vi "Read Property.vi"(8 "error in (no error)":errorcluster, 11 "2D Plot.lvclass in":refnum<class "2D Plot.lvclass">) -> (0 "error out":errorcluster, 2 "XY Graph Property Cluster":T1, 3 "2D Plot.lvclass out":refnum<class "2D Plot.lvclass">)   [LabVIEW 2020, in "2D Plot.lvclass"]
uses:
  <vilib>/Math Plots/2D Math Plots/2D Plot/2D Plot/2D Plot.lvclass
  <vilib>/Math Plots/2D Math Plots/2D Plot/2D Plot/Typedef/Property Cluster.ctl
  <vilib>/Math Plots/2D Math Plots/2D Plot/2D Plot/Typedef/Graph General Property.ctl
  <vilib>/Math Plots/2D Math Plots/2D Plot/2D Plot/Typedef/Scale Array.ctl
  <vilib>/Math Plots/2D Math Plots/2D Plot/2D Plot/Typedef/Scale Cluster.ctl
  <vilib>/Utility/miscctls.llb/LVOffsetAndMultiplierTypeDef.ctl
  <vilib>/Math Plots/2D Math Plots/2D Plot/2D Plot/Typedef/Cursor Property.ctl
  <vilib>/Utility/miscctls.llb/LVCursorListTypeDef.ctl
  <vilib>/Utility/miscctls.llb/LVAnnotationListTypeDef.ctl
  <vilib>/Math Plots/2D Math Plots/2D Plot/2D Plot/2D Plot.lvclass/2D Plot.ctl
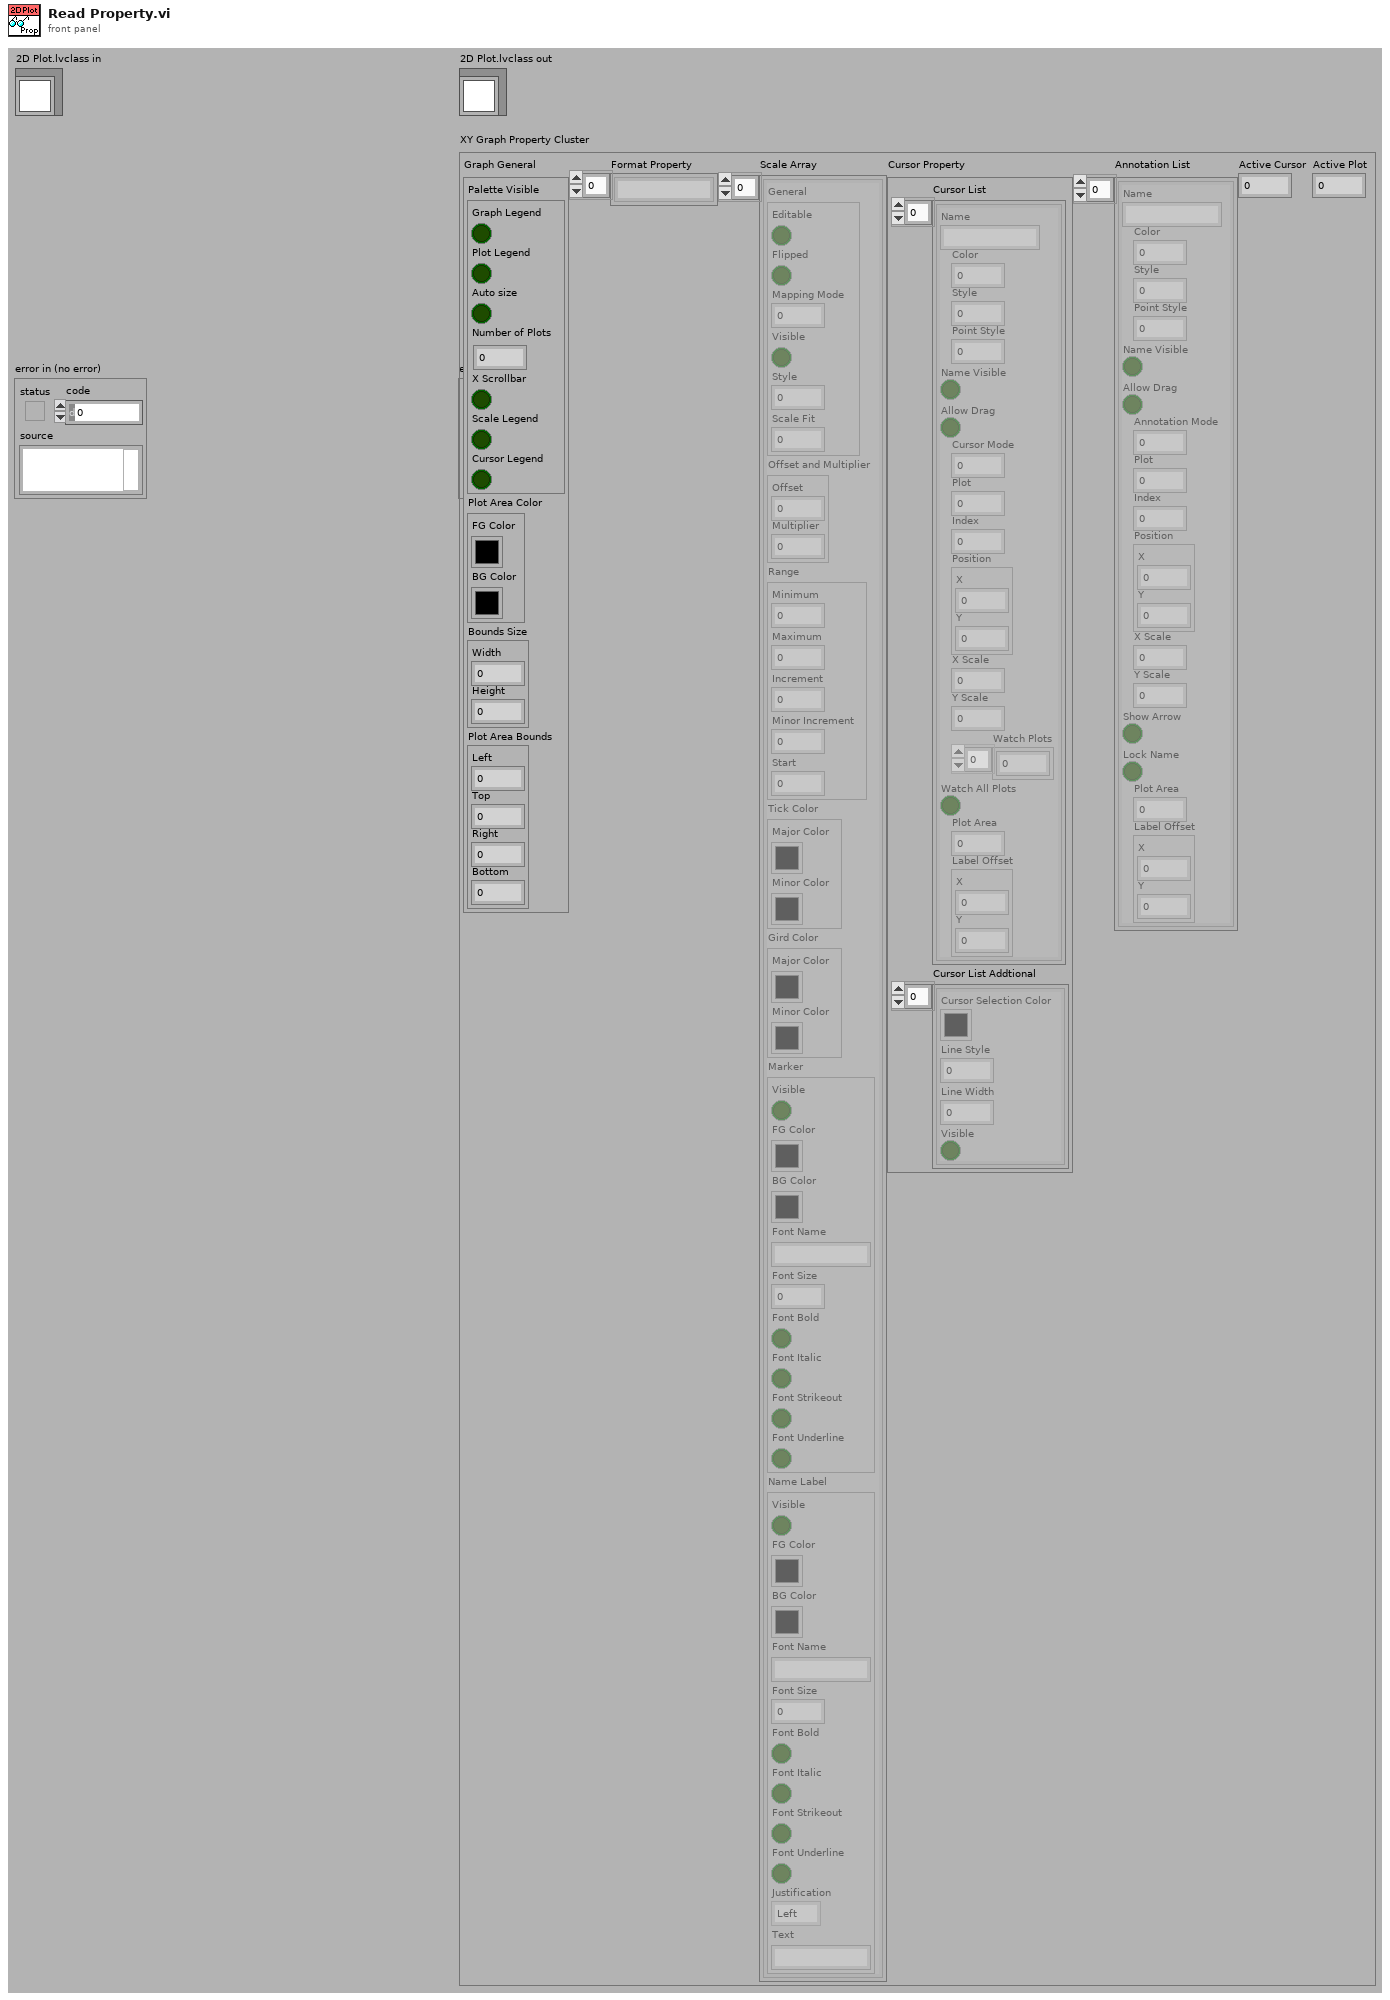
[diagram p1: front panel]
types:
  T1 = typedef "2D Plot.lvclass/Property Cluster.ctl" = cluster{"Graph General":T2, "Format Property":string[], "Scale Array":T3, "Cursor Property":T6, "Annotation List":T8, "Active Cursor":i32, "Active Plot":i32}
  T2 = typedef "2D Plot.lvclass/Graph General Property.ctl" = cluster{"Palette Visible":cluster{"Graph Legend":bool, "Plot Legend":bool, "Auto size":bool, "Number of Plots":u32, "X Scrollbar":bool, "Scale Legend":bool, "Cursor Legend":bool}, "Plot Area Color":cluster{"FG Color":u32, "BG Color":u32}, "Bounds Size":cluster{"Width":u32, "Height":u32}, "Plot Area Bounds":cluster{"Left":i16, "Top":i16, "Right":i16, "Bottom":i16}}
  T3 = typedef "2D Plot.lvclass/Scale Array.ctl" = T4[]
  T4 = typedef "2D Plot.lvclass/Scale Cluster.ctl" = cluster{"General":cluster{"Editable":bool, "Flipped":bool, "Mapping Mode":u8, "Visible":bool, "Style":u8, "Scale Fit":u8}, "Offset and Multiplier":T5, "Range":cluster{"Minimum":dbl, "Maximum":dbl, "Increment":dbl, "Minor Increment":dbl, "Start":dbl}, "Tick Color":cluster{"Major Color":u32, "Minor Color":u32}, "Gird Color":cluster{"Major Color":u32, "Minor Color":u32}, "Marker":cluster{"Visible":bool, "FG Color":u32, "BG Color":u32, "Font Name":string, "Font Size":u32, "Font Bold":bool, "Font Italic":bool, "Font Strikeout":bool, "Font Underline":bool}, "Name Label":cluster{"Visible":bool, "FG Color":u32, "BG Color":u32, "Font Name":string, "Font Size":u32, "Font Bold":bool, "Font Italic":bool, "Font Strikeout":bool, "Font Underline":bool, "Justification":enum16{"Left", "Center", "Right"}, "Text":string}}
  T5 = typedef "LVOffsetAndMultiplierTypeDef.ctl" = cluster{"Offset":dbl, "Multiplier":dbl}
  T6 = typedef "2D Plot.lvclass/Cursor Property.ctl" = cluster{"Cursor List":T7, "Cursor List Addtional":cluster{"Cursor Selection Color":u32, "Line Style":u8, "Line Width":u8, "Visible":bool}[]}
  T7 = typedef "LVCursorListTypeDef.ctl" = cluster{"Name":string, "Color":u32, "Style":u8, "Point Style":u8, "Name Visible":bool, "Allow Drag":bool, "Cursor Mode":u32, "Plot":i32, "Index":i32, "Position":cluster{"X":dbl, "Y":dbl}, "X Scale":u32, "Y Scale":u32, "Watch Plots":i32[], "Watch All Plots":bool, "Plot Area":i32, "Label Offset":cluster{"X":dbl, "Y":dbl}}[]
  T8 = typedef "LVAnnotationListTypeDef.ctl" = cluster{"Name":string, "Color":u32, "Style":u8, "Point Style":u8, "Name Visible":bool, "Allow Drag":bool, "Annotation Mode":u32, "Plot":i32, "Index":i32, "Position":cluster{"X":dbl, "Y":dbl}, "X Scale":u32, "Y Scale":u32, "Show Arrow":bool, "Lock Name":bool, "Plot Area":i32, "Label Offset":cluster{"X":dbl, "Y":dbl}}[]
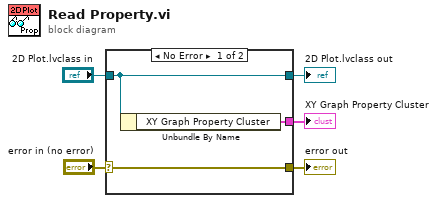
[diagram p0: block diagram]
diagram:
  n1 = case shown="No Error" "error in (no error)" {
    selector: "error in (no error)" -> [w8 w9]
    tunnel: [w8 w9] -> w4
    tunnel: [w7 w10] -> w2
    tunnel: "2D Plot.lvclass in" -> [w7 w10]
    tunnel: [w6 _] -> w1
    frame No Error {
      n2 = Unbundle By Name(w7) -> ("XY Graph Property Cluster"=w6:T1)
    }
    frame Error {
    }
  }
  "error out" <- w4
  "2D Plot.lvclass out" <- w2
  "XY Graph Property Cluster" <- w1
